vi "kebab-case Converter.vi"(4 "Input string":string) -> (1 "Output string":string)   [LabVIEW 2025, in "Name Formatter.lvlib"]
doc: "Description:\nTransforms a text with words separated by spaces into <b>kebab-case</b>. All letters are lowercase, and spaces are replaced with hyphens.\n\nExample:\nInput -> hello cruel cruel\nOutput -> helloCruelWorld\n\nRequirements:\nThe input must contain spaces. Without spaces, this conversion cannot be applied."
uses:
  Name Formatter.lvlib
panel:
  # "text with spaces"
  # "kebab-case"
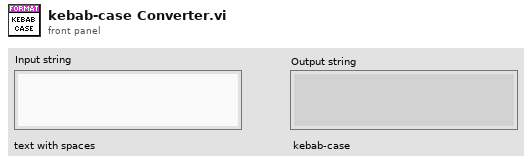
[diagram p1: front panel]
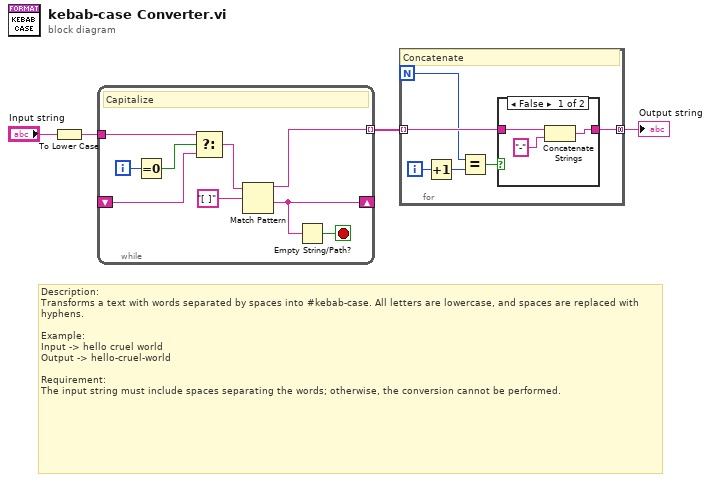
[diagram p0: block diagram]
diagram:
  # "Description:\nTransforms a text with words separated by spaces into #kebab-case. All letters are lowercase, and spaces are replaced with hyphens.\n\nExample:\nInput -> hello cruel world\nOutput -> hello-cruel-world\n\nRequirement:\nThe input string must include spaces separating the words; otherwise, the conversion cannot be performed."
  n1 = To Lower Case(string="Input string") -> (all lower case string=w1:string)
  n2 = while {
    tunnel: w1 -> [w12]
    tunnel: [w5] -> w3 mode=indexing
    shift-right: [w9] -> _
    shift-left: _ -> [w10]
    i -> [w7]
    stop <- w8 stop-if-true
    # "Capitalize"
    n3 = Equal To 0?(x=w7) -> (x = 0?=w6:bool)
    n4 = Select(t=w12, s=w6, f=w10) -> (s? t:f=w11:string)
    n5 = Match Pattern(string=w11, regular expression="[ ]") -> (before substring=w5:string, after substring=w9:string)  [unwired: 1 in, 2 out]
    n6 = Empty String/Path?(string/path=w9) -> (empty?=w8:bool)
  }
  n7 = for {
    N -> [w16]
    tunnel: w3 -> [w19] mode=indexing
    tunnel: [w18] -> w2 mode=concatenating
    i -> [w17]
    # "Concatenate"
    n8 = Increment(x=w17) -> (x+1=w15:i32)
    n9 = Equal?(x=w16, y=w15) -> (x = y?=w14:bool)
    n10 = case shown="False" w14 {
      tunnel: w19 -> [w22 w23]
      tunnel: [w20 w23] -> w18
      frame False {
        n11 = Concatenate Strings(w22, "-") -> (w20:string)
      }
      frame True {
      }
    }
  }
  "Output string" <- w2
